vi "Operation Stop.vi"(8 "error in (no error)":errorcluster, 11 "Superior Actor in":refnum<class "Node Actor.lvclass">) -> (0 "error out":errorcluster, 3 "Superior Actor out":refnum<class "Node Actor.lvclass">)   [LabVIEW 2024, in "Node Actor.lvclass"]
uses:
  Node Actor.lvclass
  C:/Users/iio/Desktop/Bussiness/Tricorn Re/Madelbrot 4.0/General Library/Ancestor Class/Actor/System Actor/System Actor.lvclass
  Node Actor.lvclass/Node Actor.ctl
  System Actor/System Actor.lvclass
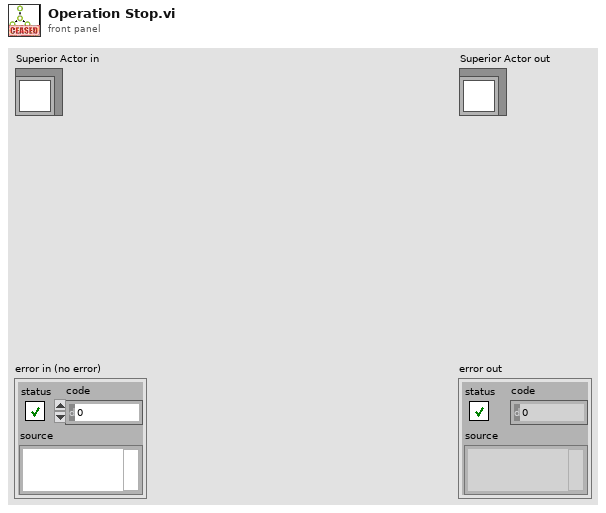
[diagram p1: front panel]
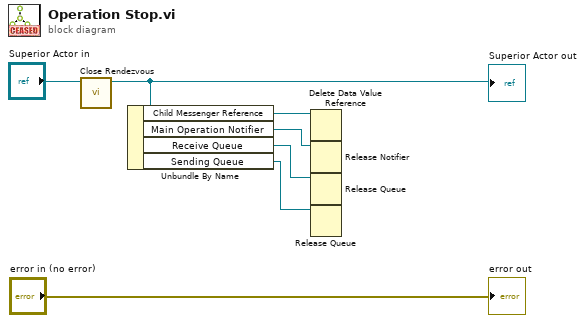
[diagram p0: block diagram]
diagram:
  n1 = call "Close Rendezvous.vi"("System Actor in"="Superior Actor in") -> ("System Actor out"=w1:refnum<class "Node Actor.lvclass">)  [unwired: 9 in, 1 out]
  "Superior Actor out" <- w1
  n2 = Unbundle By Name(w1) -> ("Child Messenger Reference"=w6:refnum<data-value>, "Main Operation Notifier"=w5:refnum<notifier>, "Receive Queue"=w4:refnum<queue>, "Sending Queue"=w3:refnum<queue>)
  n3 = Delete Data Value Reference(data value reference=w6) -> ()  [unwired: 1 in, 2 out]
  n4 = Release Notifier(notifier=w5) -> ()  [unwired: 2 in, 3 out]
  n5 = Release Queue(queue=w4) -> ()  [unwired: 2 in, 3 out]
  n6 = Release Queue(queue=w3) -> ()  [unwired: 2 in, 3 out]
  "error out" <- "error in (no error)"
